vi "Lock Publication.vi"(4 "Return Error Transport":refnum<class "ITransport.lvclass">, 6 "Publisher ID":string, 7 "PublicationPolicy":refnum<class "IPublicationPolicy.lvclass">, 8 "error in (no error)":errorcluster, 9 "Datum Type":variant, 10 "Datum Name":string, 11 "Mediator In":refnum<class "Mediator.lvclass">) -> (0 "error out":errorcluster, 3 "Mediator Out":refnum<class "Mediator.lvclass">)   [LabVIEW 2020, in "MVA Framework.lvlib" / "Mediator.lvlib" / "Mediator.lvclass"]
doc: "<License>\nCopyright © 2017 Composed Systems, LLC | All rights reserved\nwww.composed.io\n\nAuthor: Ethan Stern <ethan.stern@composed.io>\n\nThis software is provided \"AS IS\" WITHOUT WARRANTIES, either express or implied, AND IS FOR EDUCATIONAL PURPOSES ONLY.\n</License>"
uses:
  Mediator.lvclass
  composed-transport/Source/ITransport/ITransport.lvclass
  IMediator/IPublicationPolicy/IPublicationPolicy.lvclass
  Mediator.lvclass/Mediator.ctl
  TopicLookupTable/TopicLookupTable.lvclass/TopicLookupTable.ctl
  Topic Messages/Lock Topic Msg/Lock Topic Msg.lvclass/Lock Topic Msg.ctl
  <vilib>/ActorFramework/Message Enqueuer/Message Enqueuer.lvclass/Message Enqueuer.ctl
  <vilib>/ActorFramework/Message Enqueuer/Enqueue.vi
  Topic Messages/Lock Topic Msg/Lock Topic Msg.lvclass
  C:/Program Files/National Instruments/LabVIEW 2020/vi.lib/ActorFramework/Message/Message.lvclass
  variant-extensions/Source/Format Type String.vi
  <vilib>/ActorFramework/Message Priority Queue/Priority Enqueue.vi
  <vilib>/ActorFramework/Message Enqueuer/Message Enqueuer.lvclass
  TopicLookupTable/TopicLookupTable.lvclass
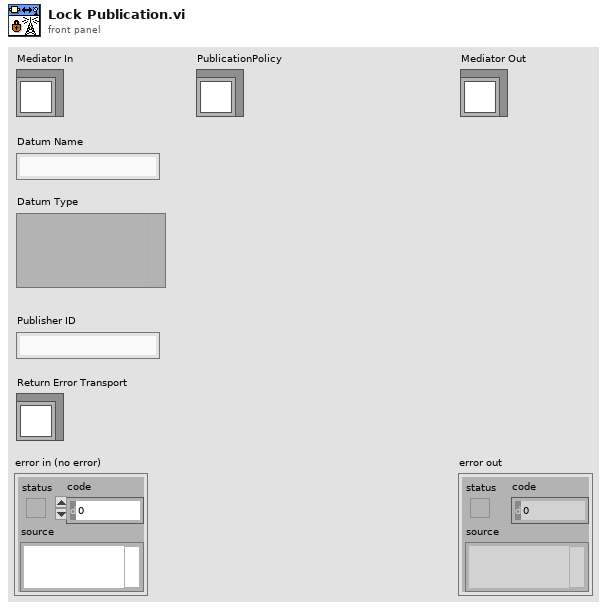
[diagram p1: front panel]
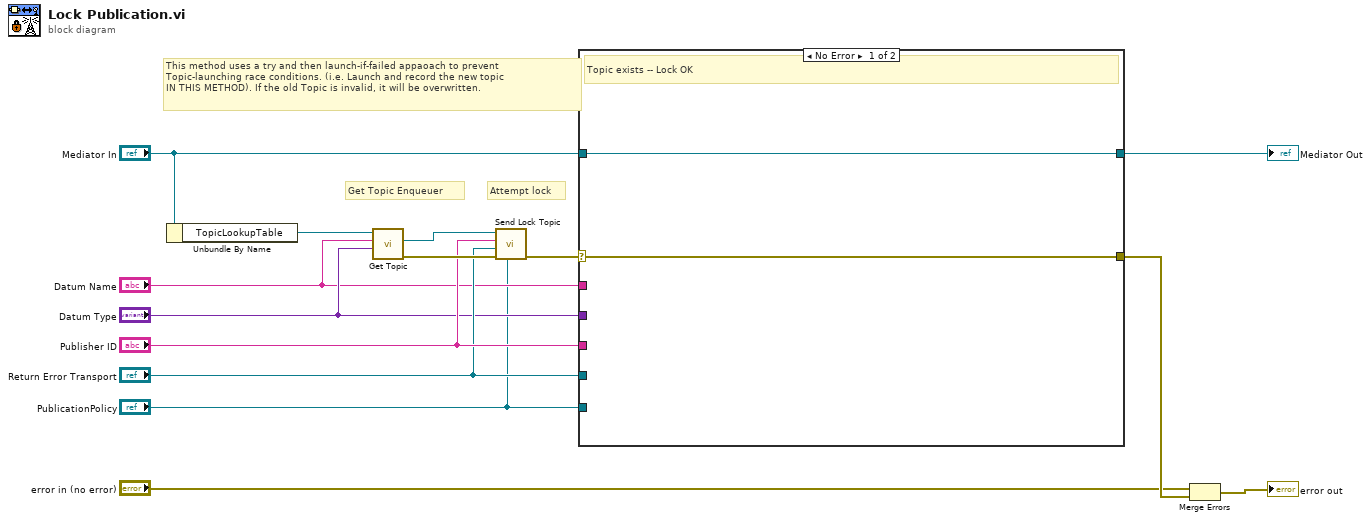
[diagram p0: block diagram]
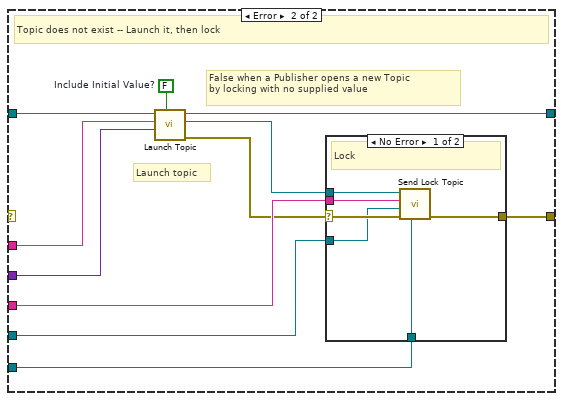
[diagram p2: hidden frame]
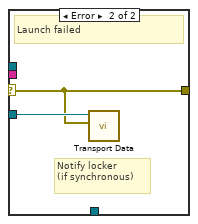
[diagram p3: hidden frame]
diagram:
  # "This method uses a try and then launch-if-failed appaoach to prevent\nTopic-launching race conditions. (i.e. Launch and record the new topic\nIN THIS METHOD). If the old Topic is invalid, it will be overwritten."
  # "Attempt lock"
  # "Get Topic Enqueuer"
  n1 = Unbundle By Name("Mediator In") -> ("TopicLookupTable"=w14:refnum<data-value>)
  n2 = call "Get Topic.vi"("Topic Type"="Datum Type", "Topic Name"="Datum Name", "TopicLookupTable"=w14) -> ("error out"=w12:errorcluster, "Topic Enqueuer"=w13:refnum<class "Message Enqueuer.lvclass">)  [unwired: 6 in, 1 out]
  n3 = call "Send Lock Topic.vi"("PublicationPolicy"="PublicationPolicy", "error in (no error)"=w12, "Return Error Transport"="Return Error Transport", "Publisher ID"="Publisher ID", "Message Enqueuer"=w13) -> ("error out"=w8:errorcluster)  [unwired: 5 in, 1 out]
  n4 = case shown="No Error" w8 {
    selector: w8 -> [w15 _]
    tunnel: "Mediator In" -> [w16 w27]
    tunnel: [w16 w25] -> w6
    tunnel: "Datum Name" -> [_ w23]
    tunnel: "Datum Type" -> [_ w22]
    tunnel: [w15 w26] -> w11
    tunnel: "Publisher ID" -> [_ w20]
    tunnel: "Return Error Transport" -> [_ w17]
    tunnel: "PublicationPolicy" -> [_ w19]
    frame No Error {
      # "Topic exists -- Lock OK"
    }
    frame Error {
      w21 = FALSE  # Include Initial Value?
      # "False when a Publisher opens a new Topic\nby locking with no supplied value"
      # "Launch topic"
      # "Topic does not exist -- Launch it, then lock"
      n5 = call-dynamic "Launch Topic.vi"("Include Initial Value? (F)"=w21, "Type"=w22, "Datum Name"=w23, "Mediator in"=w27) -> ("error out"=w18:errorcluster, "New Topic Enqueuer"=w24:refnum<class "Message Enqueuer.lvclass">, "Mediator out"=w25:refnum<class "Mediator.lvclass">)  [unwired: 5 in]
      n6 = case shown="No Error" w18 {
        selector: w18 -> [w29 w34]
        tunnel: [w33 w34] -> w26
        tunnel: w24 -> [w32 _]
        tunnel: w20 -> [w31 _]
        tunnel: w19 -> [w30 _]
        tunnel: w17 -> [w28 w35]
        frame No Error {
          # "Lock"
          n7 = call "Send Lock Topic.vi"("PublicationPolicy"=w30, "error in (no error)"=w29, "Return Error Transport"=w28, "Publisher ID"=w31, "Message Enqueuer"=w32) -> ("error out"=w33:errorcluster)  [unwired: 5 in, 1 out]
        }
        frame Error {
          # "Notify locker\n(if synchronous)"
          # "Launch failed"
          n8 = call "Transport Data.vi"("Value"=w34, "ITransport in"=w35) -> ()  [unwired: 8 in, 2 out]
        }
      }
    }
  }
  "Mediator Out" <- w6
  n9 = Merge Errors("error in (no error)", w11) -> (→"error out":errorcluster)
